vi "Read_Instr.vi"(8 "error in (no error)":errorcluster caption="entrée d'erreur (pas d'erreur)", 11 "Class DIO en entrée":refnum<class "Class Instrument DIO.lvclass">) -> (0 "error out":errorcluster caption="sortie d'erreur", 3 "Class DIO en Sortie":refnum<class "Class Instrument DIO.lvclass">)   [LabVIEW 2020, in "Library Instrument & Equipement.lvlib" / "Library Instruments.lvlib" / "Class Instrument DIO.lvclass"]
uses:
  Class Instrument DIO.lvclass
  Class Instrument DIO.lvclass/Class Instrument DIO.ctl
  Instrument (Default)/Class Instrument (Default).lvclass
  DIO/Class DIO (Default)/Class DIO (Default).lvclass
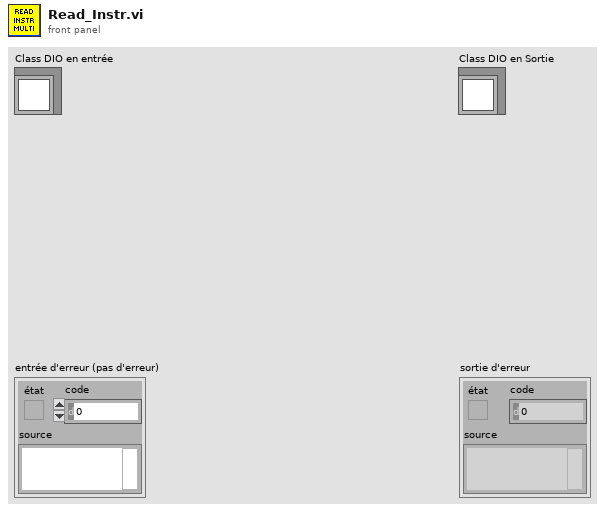
[diagram p1: front panel]
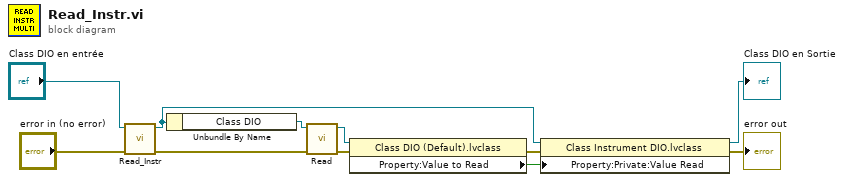
[diagram p0: block diagram]
diagram:
  n1 = call-parent "Read_Instr.vi"("error in (no error)"="error in (no error)", "Class Instrument (Default) en entrée"="Class DIO en entrée") -> ("error out"=w3:errorcluster, "Class Instrument (Default) en sortie"=w9:refnum<class "Class Instrument DIO.lvclass">)  [unwired: 8 in]
  n2 = Unbundle By Name(w9) -> ("Class DIO"=w4:refnum<class "Class DIO (Default).lvclass">)
  n3 = call-dynamic "Read.vi"("error in (no error)"=w3, "Class DIO (Default) en entrée"=w4) -> ("error out"=w2:errorcluster, "Class DIO (Default) en sortie"=w1:refnum<class "Class DIO (Default).lvclass">)  [unwired: 8 in]
  n4 = property class="Class DIO (Default).lvclass"(reference=w1, error in=w2) -> (error out=w7:errorcluster, "Property:Value to Read"=w5:bool)  [unwired: 1 out]
  n5 = property class="Class Instrument DIO.lvclass"(reference=w9, error in=w7, "Property:Private:Value Read"=w5) -> (reference out=→"Class DIO en Sortie":refnum<class "Class Instrument DIO.lvclass">, error out=→"error out":errorcluster)
